vi "Terminate ssh-agent.vi"(8 "error in (no error)":errorcluster, 11 "Agent Fixture in":refnum<class "Agent Fixture.lvclass">) -> (0 "error out":errorcluster, 1 "Standard Error":string, 2 "Standard Output":string, 3 "Agent Fixture out":refnum<class "Agent Fixture.lvclass">)   [LabVIEW 2013, in "libssh2_integration_tests.lvlib" / "Agent Fixture.lvclass"]
uses:
  Agent Fixture.lvclass
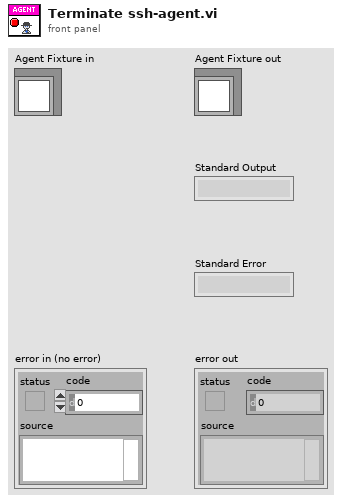
[diagram p1: front panel]
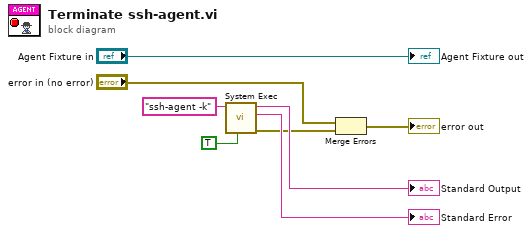
[diagram p0: block diagram]
diagram:
  n1 = call <vilib>:"System Exec.vi"("run minimized? (F)"=TRUE, "command line"="ssh-agent -k") -> ("error out"=w1:errorcluster, "standard error"=→"Standard Error":string, "standard output"=→"Standard Output":string)  [unwired: 6 in, 1 out]
  n2 = Merge Errors("error in (no error)", w1) -> (→"error out":errorcluster)
  "Agent Fixture out" <- "Agent Fixture in"
